vi "Write Writer.vi"(8 "Error In":errorcluster, 10 "Writer":refnum<class "Writer.lvclass">, 11 "Renderer In":refnum<class "Renderer.lvclass">) -> (0 "Error Out":errorcluster, 3 "Renderer Out":refnum<class "Renderer.lvclass">)   [LabVIEW 2018, in "Toolkit.lvlib" / "Renderer.lvclass"]
uses:
  Renderer.lvclass
  Writers/Writer/Writer.lvclass
  Renderer.lvclass/Renderer.ctl
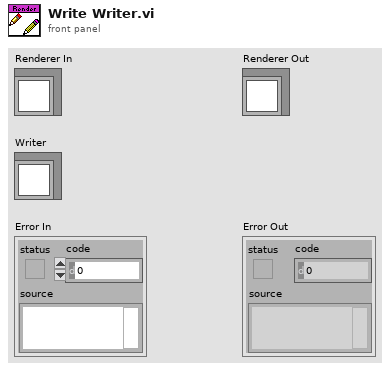
[diagram p1: front panel]
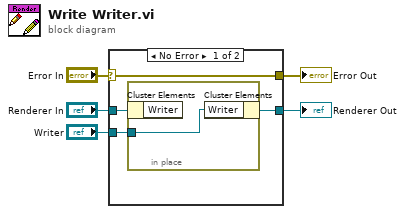
[diagram p0: block diagram]
diagram:
  n1 = case shown="No Error" "Error In" {
    selector: "Error In" -> [w9 w11]
    tunnel: [w9 w11] -> w4
    tunnel: [w7 w12] -> w2
    tunnel: "Renderer In" -> [w8 w12]
    tunnel: "Writer" -> [w6 _]
    frame No Error {
      n2 = in-place {
        in-place-border: w6 -> [w10]
        n3 = in-place-cluster #1(w8) -> ()  [unwired: 1 out]
        n4 = in-place-cluster #1("Writer"=w10) -> (w7:refnum<class "Renderer.lvclass">)
      }
    }
    frame Error {
    }
  }
  "Error Out" <- w4
  "Renderer Out" <- w2
